vi "Get Local IP.vi"(8 "error in (no error)":errorcluster) -> (0 "error out":errorcluster, 2 "Local IP":string)   [LabVIEW 2020, in "Controller.lvlib"]
uses:
  Controller.lvlib
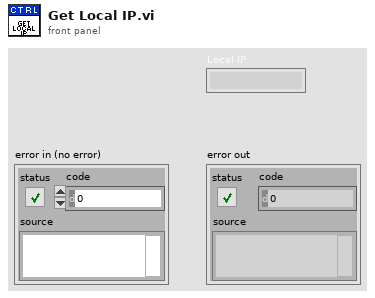
[diagram p1: front panel]
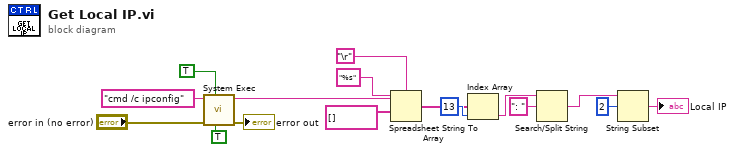
[diagram p0: block diagram]
diagram:
  n1 = call <vilib>:"System Exec.vi"("run minimized? (F)"=TRUE, "wait until completion? (T)"=TRUE, "error in (no error)"="error in (no error)", "command line"="cmd /c ipconfig") -> ("error out"=→"error out":errorcluster, "standard output"=w10:string)  [unwired: 4 in, 2 out]
  n2 = Spreadsheet String To Array(delimiter (Tab)="\r", format string="%s", spreadsheet string=w10, array type (2D Dbl)=string[] []) -> (array=w7:string[])
  n3 = Index Array(array=w7, index=13) -> (element=w6:string)
  n4 = Search/Split String(string=w6, search string/char (-)=": ") -> (match + rest of string=w5:string)  [unwired: 1 in, 2 out]
  n5 = String Subset(string=w5, offset (0)=2) -> (substring=→"Local IP":string)  [unwired: 1 in]
